vi "pharosOpen.vi"(0 "sample mode":i32(ring)=10178 items=["Finite Samples"=10178, "Continuous Samples"=10123, "Hardware Timed Single Point"=12522]) -> ()   [LabVIEW 2017]
uses:
  globalDevices.vi
  <vilib>/DAQmx/create/channels.llb/DAQmx Create Channel (DO-Digital Output).vi
  <vilib>/DAQmx/configure/timing.llb/DAQmx Timing (Sample Clock).vi
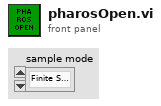
[diagram p1: front panel]
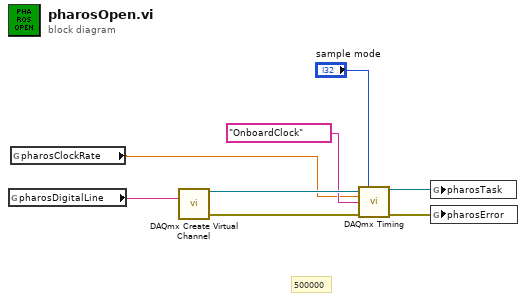
[diagram p0: block diagram]
diagram:
  # "500000"
  n1 = global read "globalDevices.vi" "pharosDigitalLine"() -> (w4:tag)
  n2 = global read "globalDevices.vi" "pharosClockRate"() -> (w1:dbl)
  n3 = call-poly <vilib>:"DAQmx Create Virtual Channel.vi"("lines"=w4) -> ("task out"=w8:refnum<k21>, "error out"=w5:errorcluster)  [unwired: 13 in]
  n4 = call-poly <vilib>:"DAQmx Timing.vi"("task/channels in"=w8, "sample mode"="sample mode", "rate"=w1, "source"=tag "OnboardClock", "error in"=w5) -> ("task out"=w3:refnum<k21>, "error out"=w2:errorcluster)  [unwired: 9 in]
  n5 = global write "globalDevices.vi" "pharosTask"(w3) -> ()
  n6 = global write "globalDevices.vi" "pharosError"(w2) -> ()
